vi "F Dwf Digital Spi Write32.vi"(6 "cTX":i32, 7 "rgTX":u32, 8 "error in (no error)":errorcluster, 9 "cBitPerWord":i32, 10 "cDQ":i32, 11 "hdwf":i32) -> (0 "error out":errorcluster, 3 "function return":i32, 5 "rgTX out":u32)   [LabVIEW 2021, in "Olasdwf.lvlib"]
doc: "DWFAPI int FDwfDigitalSpiWrite32(HDWF hdwf, int cDQ, int cBitPerWord, unsigned int *rgTX, int cTX);"
uses:
  Olasdwf.lvlib
  Windows/System32/dwf.dll
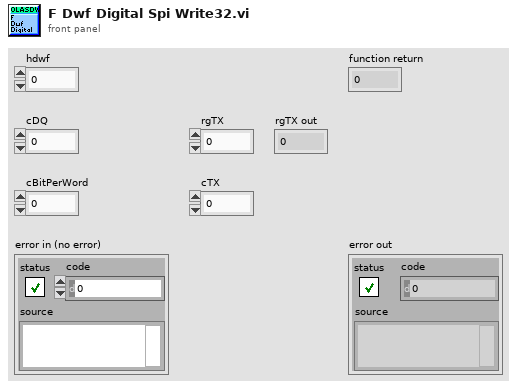
[diagram p1: front panel]
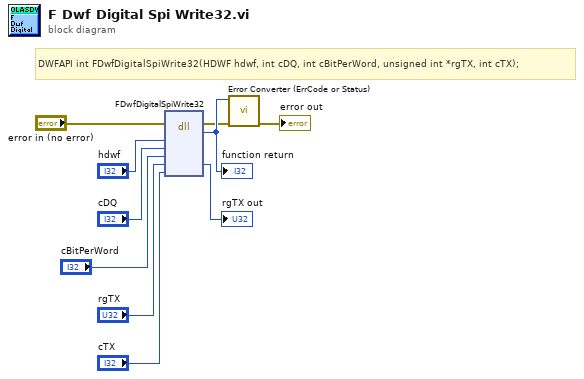
[diagram p0: block diagram]
diagram:
  # "DWFAPI int FDwfDigitalSpiWrite32(HDWF hdwf, int cDQ, int cBitPerWord, unsigned int *rgTX, int cTX);"
  n1 = dll-call lib="/Windows/System32/dwf.*" fn="FDwfDigitalSpiWrite32"(error in="error in (no error)", "hdwf"="hdwf", "cDQ"="cDQ", "cBitPerWord"="cBitPerWord", "rgTX"="rgTX", "cTX"="cTX") -> (error out=w2:errorcluster, w10:i32, "rgTX"=→"rgTX out":u32)  [unwired: 6 in, 1 out]
  "function return" <- w10
  n2 = call "Error Converter (ErrCode or Status).vi"("error in (no error)"=w2, "error code"=w10) -> ("error out"=→"error out":errorcluster)  [unwired: 9 in]
